vi "Server - Test Outbound Traffic from Server.vi"(8 "error in (no error)":errorcluster, 11 "ports to check":u16[](array[numeric])=[82, 482, 5672, 6343, 8002, 49580, 3580, 80, 22, 44516, 52725, 8080]) -> (0 "error out":errorcluster, 2 "log file path":path, 3 "Results":string[][](array[string]))   [LabVIEW 2019]
doc: "Demonstrates how to set up a basic TCP connection, send data to the specified port once a connection has been established, and terminate the connection once the data has been sent. This VI is designed to stop if the TCP connection is terminated. The data sent in this example is an array of random numbers."
panel:
  out "log file name":string
  out "current test":cluster{string, "error out":errorcluster}
  in  "Start test":bool
  out "current port":u16
  out "Waveform Graph":dbl[](graph)
  # "1. Run the executable\n2. Open and run the Test Server Outboun Client PC on the client computer and follow the instructions on its front panel. Note that if you wait longer than 60 seconds to do this after running this VI, it will time out.\n3. Click on the button Start Test\n4. Click Stop to stop the VI. Note that if you stop the client VI, this VI will stop automatically."
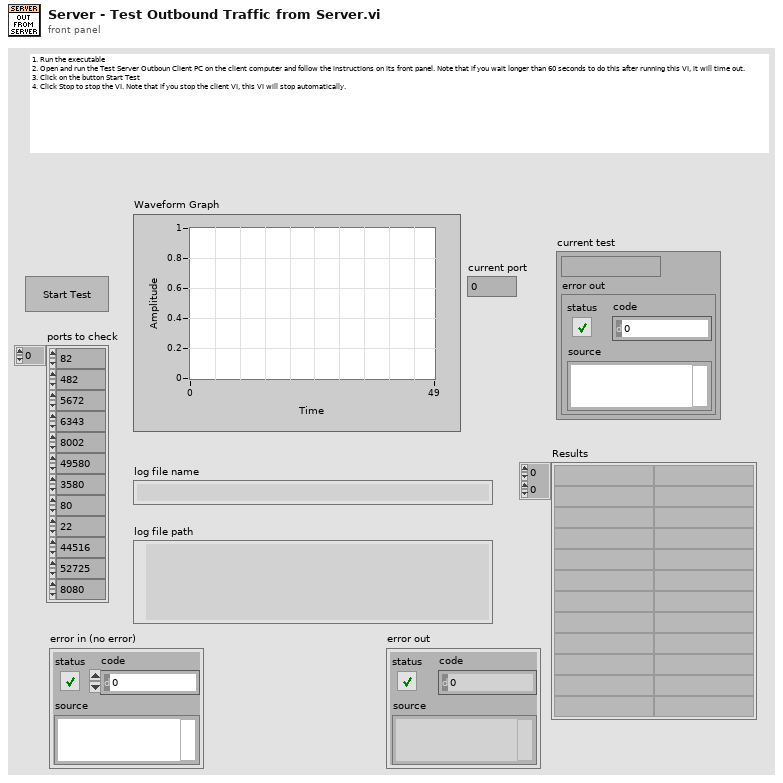
[diagram p1: front panel]
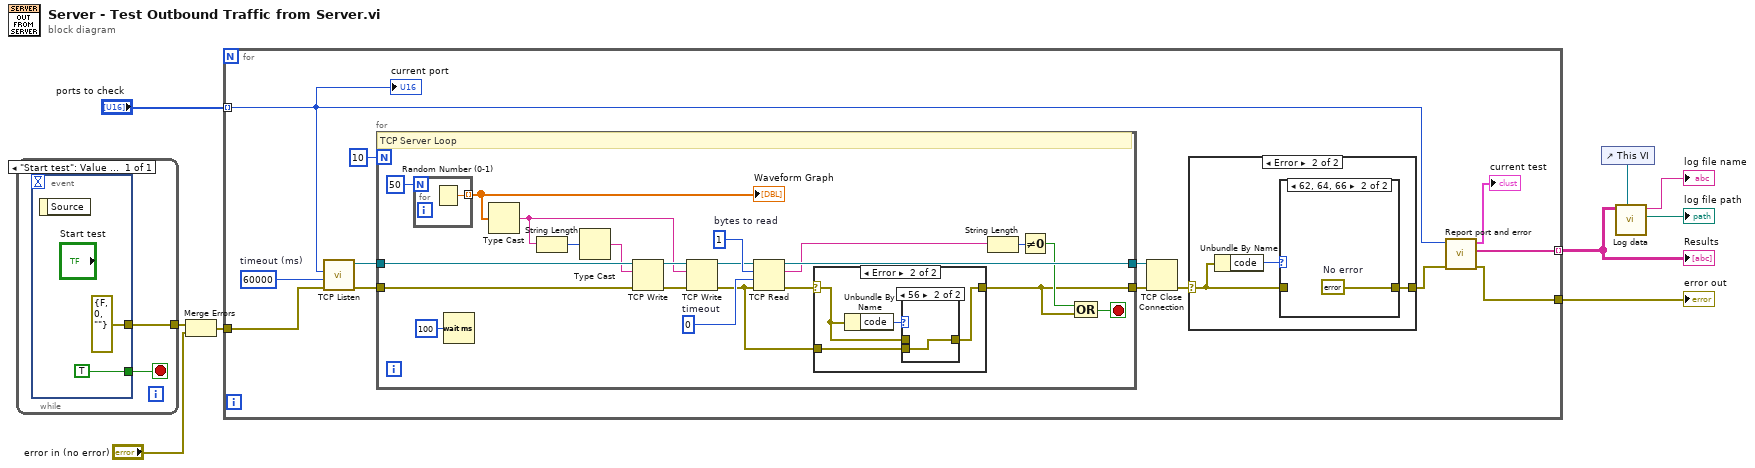
[diagram p0: block diagram]
diagram:
  n1 = while {
    tunnel: [w11] -> w3
    stop <- w10 stop-if-true
    n2 = event shown="[0] \"Start test\": Value Change" {
      selector: _ -> [_]
      dyn-events: _ -> [_]
      timeout: _ -> [_]
      tunnel: [errorcluster {"status"=FALSE, "code"=0, "source"=""} ("error constant")] -> w11
      tunnel: [TRUE] -> w10
      event "Start test": Value Change {
        n3 = event-data() -> ()  [unwired: 1 in, 1 out]
      }
    }
  }
  n4 = Merge Errors(w3, "error in (no error)") -> (w2:errorcluster)
  n5 = for {
    tunnel: "ports to check" -> [w20] mode=indexing
    tunnel: [w17] -> w8 mode=indexing
    tunnel: w2 -> [w15]
    tunnel: [w14] -> w1
    w21 = 60000  # timeout (ms)
    n6 = call <vilib>:"TCP Listen.vi"("error in (no error)"=w15, "timeout ms (wait forever: -1)"=w21, "port"=w20) -> ("error out"=w22:errorcluster, "connection ID"=w23:refnum<k5>)  [unwired: 4 in, 3 out]
    n7 = for {
      N: 10 -> [_]
      tunnel: [w29] -> w25
      tunnel: [w35] -> w26
      tunnel: w23 -> [w47]
      tunnel: w22 -> [w39]
      stop <- w27 stop-if-true
      w34 = 0  # timeout
      w37 = 1  # bytes to read
      # "TCP Server Loop"
      n8 = for {
        N: 50 ("# of Points") -> [_]
        tunnel: [w55] -> w38 mode=indexing
        n9 = Random Number (0-1)() -> (number: 0 to 1=w55:dbl)
      }
      "Waveform Graph" <- w38
      n10 = Wait (ms)(milliseconds to wait=u32 100) -> ()  [unwired: 1 out]
      n11 = Type Cast(x=w38) -> (*(type *) &x=w42:string)  [unwired: 1 out]
      n12 = String Length(string=w42) -> (length=w44:i32)
      n13 = Type Cast(x=w44) -> (*(type *) &x=w43:string)  [unwired: 1 out]
      n14 = TCP Write(connection ID=w47, data in=w43, error in (no error)=w39) -> (connection ID out=w46:refnum<k5>, error out=w45:errorcluster)  [unwired: 2 out]
      n15 = TCP Write(connection ID=w46, data in=w42, error in (no error)=w45) -> (connection ID out=w36:refnum<k5>, error out=w28:errorcluster)  [unwired: 2 out]
      n16 = TCP Read(connection ID=w36, bytes to read=w37, error in (no error)=w28, 9:w34) -> (connection ID out=w35:refnum<k5>, data out=w32:string, error out=w30:errorcluster)  [unwired: 1 out]
      n17 = case shown="Error" w30 {
        selector: w30 -> [w48 w51]
        tunnel: [w48 w49] -> w29
        tunnel: w28 -> [_ w50]
        frame No Error {
        }
        frame Error {
          n18 = Unbundle By Name(w51) -> ("code"=w52:i32)
          n19 = case shown="56" w52 {
            tunnel: w51 -> [w53 _]
            tunnel: w50 -> [_ w54]
            tunnel: [w53 w54] -> w49
            frame Default {
            }
            frame 56 {
            }
          }
        }
      }
      n20 = String Length(string=w32) -> (length=w33:i32)
      n21 = Not Equal To 0?(x=w33) -> (x != 0?=w31:bool)
      n22 = Compound Arithmetic op=OR(w31, w29) -> (w27:bool)
    }
    n23 = TCP Close Connection(connection ID=w26, error in (no error)=w25) -> (error out=w24:errorcluster)  [unwired: 2 out]
    n24 = case shown="Error" w24 {
      selector: w24 -> [w56 w58]
      tunnel: [w56 w57] -> w19
      frame No Error {
      }
      frame Error {
        n25 = Unbundle By Name(w58) -> ("code"=w59:i32)
        n26 = case shown="62, 64, 66" w59 {
          tunnel: w58 -> [w60 _]
          tunnel: [w60 w61] -> w57
          frame Default {
          }
          frame 62, 64, 66 {
            w61 = errorcluster {"status"=FALSE, "code"=0, "source"=""}  # No error
          }
        }
      }
    }
    n27 = call "Report port and error.vi"("error in (no error)"=w19, "port"=w20) -> ("error out"=w14:errorcluster, "Array"=w17:string[], "output cluster"=→"current test":cluster{string, "error out":errorcluster})  [unwired: 7 in]
    "current port" <- w20
  }
  "Results" <- w8
  "error out" <- w1
  n28 = control-ref of="This VI"() -> (w5:refnum<vi>)
  n29 = call "Log data.vi"("reference"=w5, "Data"=w8) -> ("log file path"=→"log file path":path, "log file name"=→"log file name":string)  [unwired: 7 in, 1 out]
